vi "Write VI Refnum.vi"(8 "error in (no error)":errorcluster, 10 "VI Refnum":refnum<vi>, 11 "BD_PAPAS_USD_ING in":refnum<class "BD_PAPAS_USD_ING.lvclass">) -> (0 "error out":errorcluster, 3 "BD_PAPAS_USD_ING out":refnum<class "BD_PAPAS_USD_ING.lvclass">)   [LabVIEW 2019, in "BD_PAPAS_USD_ING.lvlib" / "BD_PAPAS_USD_ING.lvclass"]
uses:
  BD_PAPAS_USD_ING.lvclass
  BD_PAPAS_USD_ING.lvclass/BD_PAPAS_USD_ING.ctl
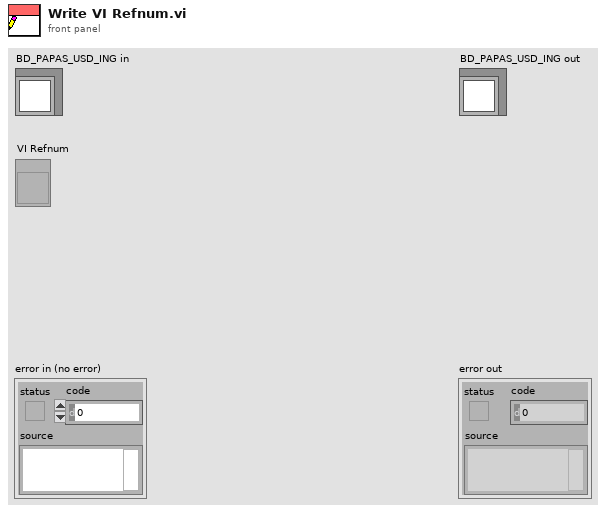
[diagram p1: front panel]
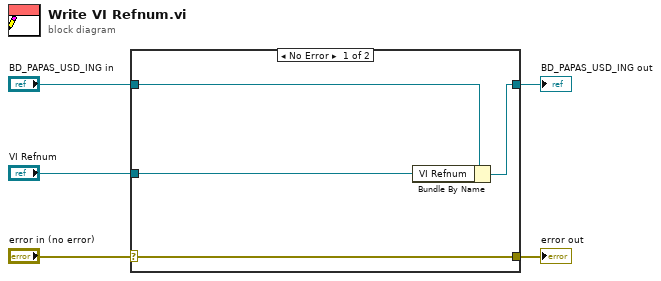
[diagram p0: block diagram]
diagram:
  n1 = case shown="No Error" "error in (no error)" {
    selector: "error in (no error)" -> [w9 w10]
    tunnel: [w9 w10] -> w4
    tunnel: [w7 w11] -> w2
    tunnel: "BD_PAPAS_USD_ING in" -> [w8 w11]
    tunnel: "VI Refnum" -> [w6 _]
    frame No Error {
      n2 = Bundle By Name(cluster=w8, "VI Refnum"=w6) -> (w7:refnum<class "BD_PAPAS_USD_ING.lvclass">)
    }
    frame Error {
    }
  }
  "error out" <- w4
  "BD_PAPAS_USD_ING out" <- w2
